vi "Configure Multi Eval Meas Limit Inband Emission IQ Offset.vi"(4 "Offset 3 (0.0)":dbl format="%^.3e", 5 "Offset 2 (0.0)":dbl format="%^.3e", 6 "Offset 1 (2.1)":dbl=2.1 format="%^.3e", 7 "Offset 0 (-2.6)":dbl=-2.6 format="%^.3e", 8 "error in (no error)":errorcluster, 9 "Modulation (Pi/2-BPSK)":i32(ring) items=["Pi/2-BPSK", "Pi/2-BPSK With Shaping", "QPSK", "16-QAM", "64-QAM", "256-QAM"], 10 "Instance (1)":T1=1, 11 "VISA resource name":refnum<visa-resource-name>) -> (0 "error out":errorcluster, 3 "VISA resource name out":refnum<visa-resource-name>)   [LabVIEW 2020, in "Rohde&Schwarz CMWXP NR FR1 Measurement.lvlib"]
doc: "Defines I/Q origin offset values used for calculation of an upper limit for the inband emission. Four different values can be set for four TX power ranges.\n\nAttributes:\nRSCMWXPNRFR1M_ATTR_MULTI_EVAL_MEAS_LIMIT_PI_2_INBAND_EMISSION_IQ_OFFSET\nRSCMWXPNRFR1M_ATTR_MULTI_EVAL_MEAS_LIMIT_BPSK_SHAPING_INBAND_EMISSION_IQ_OFFSET\nRSCMWXPNRFR1M_ATTR_MULTI_EVAL_MEAS_LIMIT_QPSK_INBAND_EMISSION_IQ_OFFSET\nRSCMWXPNRFR1M_ATTR_MULTI_EVAL_MEAS_LIMIT_QAM_INBAND_EMISSION_IQ_OFFSET\n\nRemote-control commands:\nCONFigure:NRSub:MEAS<i>:MEValuation:LIMit:PHBPsk:IBE:IQOFfset\nCONFigure:NRSub:MEAS<i>:MEValuation:LIMit:BPWShaping:IBE:IQOFfset\nCONFigure:NRSub:MEAS<i>:MEValuation:LIMit:QPSK:IBE:IQOFfset\nCONFigure:NRSub:MEAS<i>:MEValuation:LIMit:QAM<order>:IBE:IQOFfset"
uses:
  <instrlib>/Rohde&Schwarz CMWXP NR FR1 Measurement/Rohde&Schwarz CMWXP NR FR1 Measurement.lvlib
  <instrlib>/Rohde&Schwarz CMWXP NR FR1 Measurement/Private/_Instance.ctl
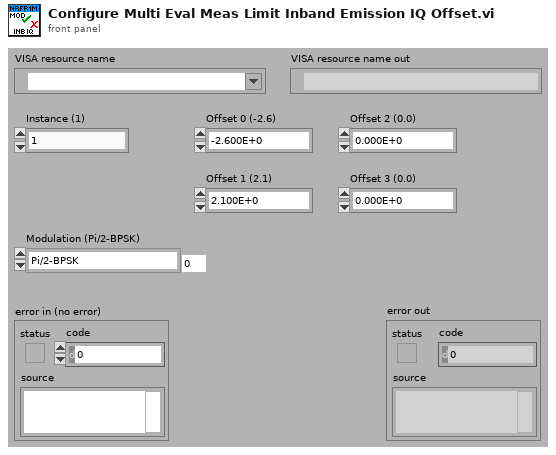
[diagram p1: front panel]
types:
  T1 = typedef "Rohde&Schwarz CMWXP NR FR1 Measurement.lvlib/_Instance.ctl" = i32
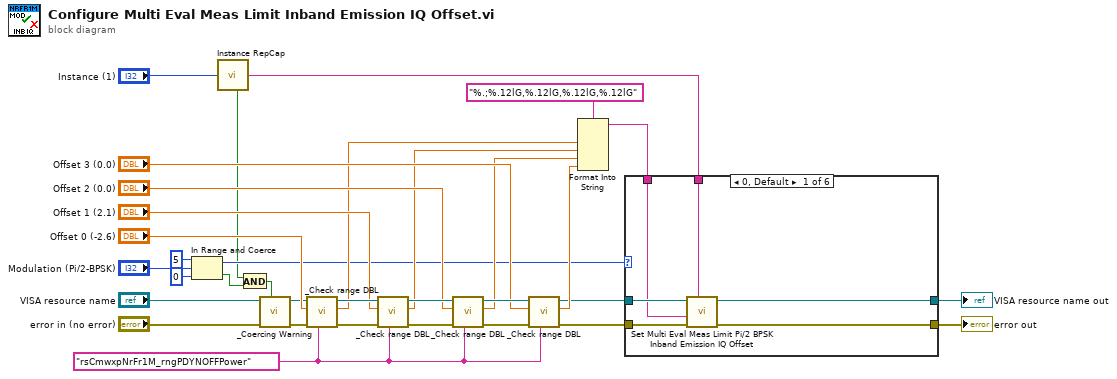
[diagram p0: block diagram]
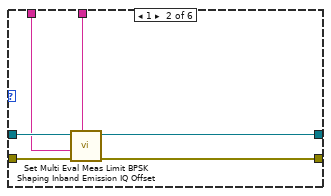
[diagram p2: hidden frame]
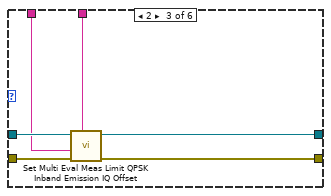
[diagram p3: hidden frame]
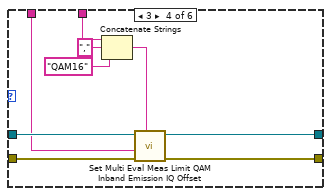
[diagram p4: hidden frame]
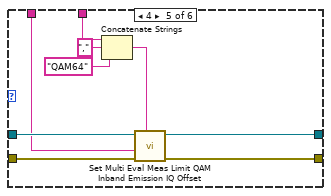
[diagram p5: hidden frame]
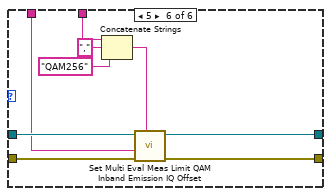
[diagram p6: hidden frame]
diagram:
  w12 = "rsCmwxpNrFr1M_rngPDYNOFFPower" ("Range Table Identifier")
  n1 = In Range and Coerce(upper limit=5, x="Modulation (Pi/2-BPSK)", lower limit=0) -> (coerced(x)=w10:i32, In Range?=w2:bool)
  n2 = call <instrlib>:"Instance RepCap.vi"("Instance In"="Instance (1)") -> ("In Range?"=w1:bool, "RepCap Identifier Out"=w31:string)  [unwired: 1 in]
  n3 = And(x=w1, y=w2) -> (x .and. y?=w3:bool)
  n4 = call <instrlib>:"_Coercing Warning.vi"("In Range?"=w3, "error in (no error)"="error in (no error)", "VISA resource name"="VISA resource name") -> ("error out"=w5:errorcluster, "VISA resource name out"=w4:refnum<visa-resource-name>)  [unwired: 7 in]
  n5 = call <instrlib>:"_Check range DBL.vi"("Range Table Identifier"=w12, "error in (no error)"=w5, "DBL Value In"="Offset 0 (-2.6)", "VISA resource name"=w4) -> ("error out"=w30:errorcluster, "DBL Value Out"=w18:dbl, "VISA resource name out"=w29:refnum<visa-resource-name>)  [unwired: 5 in]
  n6 = call <instrlib>:"_Check range DBL.vi"("Range Table Identifier"=w12, "error in (no error)"=w30, "DBL Value In"="Offset 1 (2.1)", "VISA resource name"=w29) -> ("error out"=w28:errorcluster, "DBL Value Out"=w17:dbl, "VISA resource name out"=w27:refnum<visa-resource-name>)  [unwired: 5 in]
  n7 = call <instrlib>:"_Check range DBL.vi"("Range Table Identifier"=w12, "error in (no error)"=w28, "DBL Value In"="Offset 2 (0.0)", "VISA resource name"=w27) -> ("error out"=w26:errorcluster, "DBL Value Out"=w16:dbl, "VISA resource name out"=w25:refnum<visa-resource-name>)  [unwired: 5 in]
  n8 = call <instrlib>:"_Check range DBL.vi"("Range Table Identifier"=w12, "error in (no error)"=w26, "DBL Value In"="Offset 3 (0.0)", "VISA resource name"=w25) -> ("error out"=w14:errorcluster, "DBL Value Out"=w15:dbl, "VISA resource name out"=w13:refnum<visa-resource-name>)  [unwired: 5 in]
  n9 = Format Into String(format string="%.;%.12lG,%.12lG,%.12lG,%.12lG", w18, w17, w16, w15) -> (resulting string=w20:string)  [unwired: 2 in, 1 out]
  n10 = case shown="0, Default" w10 {
    tunnel: [w40 w46 w52 w61 w70 w79] -> w34
    tunnel: [w39 w45 w51 w60 w69 w78] -> w33
    tunnel: w31 -> [w38 w44 w50 w56 w65 w74]
    tunnel: w13 -> [w37 w43 w49 w59 w68 w77]
    tunnel: w14 -> [w36 w42 w48 w58 w67 w76]
    tunnel: w20 -> [w35 w41 w47 w57 w66 w75]
    frame 0, Default {
      n11 = call "Set Multi Eval Meas Limit Pi/2 BPSK Inband Emission IQ Offset"("Repeated Capabilities"=w38, "error in (no error)"=w36, "Multi Eval Meas Limit Pi/2 BPSK Inband Emission IQ Offset ()"=w35, "instrument handle"=w37) -> ("error out"=w40:errorcluster, "instrument handle out"=w39:refnum<visa-resource-name>)  [unwired: 6 in]
    }
    frame 1 {
      n12 = call "Set Multi Eval Meas Limit BPSK Shaping Inband Emission IQ Offset"("Repeated Capabilities"=w44, "error in (no error)"=w42, "Multi Eval Meas Limit BPSK Shaping Inband Emission IQ Offset ()"=w41, "instrument handle"=w43) -> ("error out"=w46:errorcluster, "instrument handle out"=w45:refnum<visa-resource-name>)  [unwired: 6 in]
    }
    frame 2 {
      n13 = call "Set Multi Eval Meas Limit QPSK Inband Emission IQ Offset"("Repeated Capabilities"=w50, "error in (no error)"=w48, "Multi Eval Meas Limit QPSK Inband Emission IQ Offset ()"=w47, "instrument handle"=w49) -> ("error out"=w52:errorcluster, "instrument handle out"=w51:refnum<visa-resource-name>)  [unwired: 6 in]
    }
    frame 3 {
      n14 = Concatenate Strings(w56, "," ("string"), "QAM16" ("string")) -> (w53:string)
      n15 = call "Set Multi Eval Meas Limit QAM Inband Emission IQ Offset"("Repeated Capabilities"=w53, "error in (no error)"=w58, "Multi Eval Meas Limit QAM Inband Emission IQ Offset ()"=w57, "instrument handle"=w59) -> ("error out"=w61:errorcluster, "instrument handle out"=w60:refnum<visa-resource-name>)  [unwired: 6 in]
    }
    frame 4 {
      n16 = Concatenate Strings(w65, "," ("string"), "QAM64" ("string")) -> (w62:string)
      n17 = call "Set Multi Eval Meas Limit QAM Inband Emission IQ Offset"("Repeated Capabilities"=w62, "error in (no error)"=w67, "Multi Eval Meas Limit QAM Inband Emission IQ Offset ()"=w66, "instrument handle"=w68) -> ("error out"=w70:errorcluster, "instrument handle out"=w69:refnum<visa-resource-name>)  [unwired: 6 in]
    }
    frame 5 {
      n18 = Concatenate Strings(w74, "," ("string"), "QAM256" ("string")) -> (w71:string)
      n19 = call "Set Multi Eval Meas Limit QAM Inband Emission IQ Offset"("Repeated Capabilities"=w71, "error in (no error)"=w76, "Multi Eval Meas Limit QAM Inband Emission IQ Offset ()"=w75, "instrument handle"=w77) -> ("error out"=w79:errorcluster, "instrument handle out"=w78:refnum<visa-resource-name>)  [unwired: 6 in]
    }
  }
  "error out" <- w34
  "VISA resource name out" <- w33
